vi "Write General Data.vi"(8 "Error In":errorcluster, 9 "AC Advance Step Data":T1 {"Transient Time" format="%.1f ms"; "Transient Site" format="%.0f ¢X"; "Transient Volt" format="%.1f V"; "CF Lo Limit" format="%.2f"; "CF Hi Limit" format="%.2f"; "Q Lo Limit" format="%.0f VAR"; "Q Hi Limit" format="%.0f VAR"; "VA Lo Limit" format="%.0f VA"; "VA Hi Limit" format="%.0f VA"; "PF Lo Limit" format="%.3f"; "PF Hi Limit" format="%.3f"; "P Lo Limit" format="%.0f W"; "P Hi Limit" format="%.0f W"; "AP Lo Limit" format="%.1f A"; "AP Hi Limit" format="%.1f A"; "A Lo Limit" format="%.2f A"; "A Hi Limit" format="%.2f A"; "Delay Time" format="%.1f s"; "£GT" format="%.0f ms"; "£GF" format="%.1f Hz"; "£GV" format="%.1f V"; "Time" format="%.1f s"; "Voltage" format="%.1f V"; "Frequency" format="%.1f Hz"}, 10 "Modbus ID":string, 11 "VISA resource name":refnum<visa-resource-name>) -> (0 "Error Out":errorcluster, 3 "VISA resource name out":refnum<visa-resource-name>)   [LabVIEW 2013]
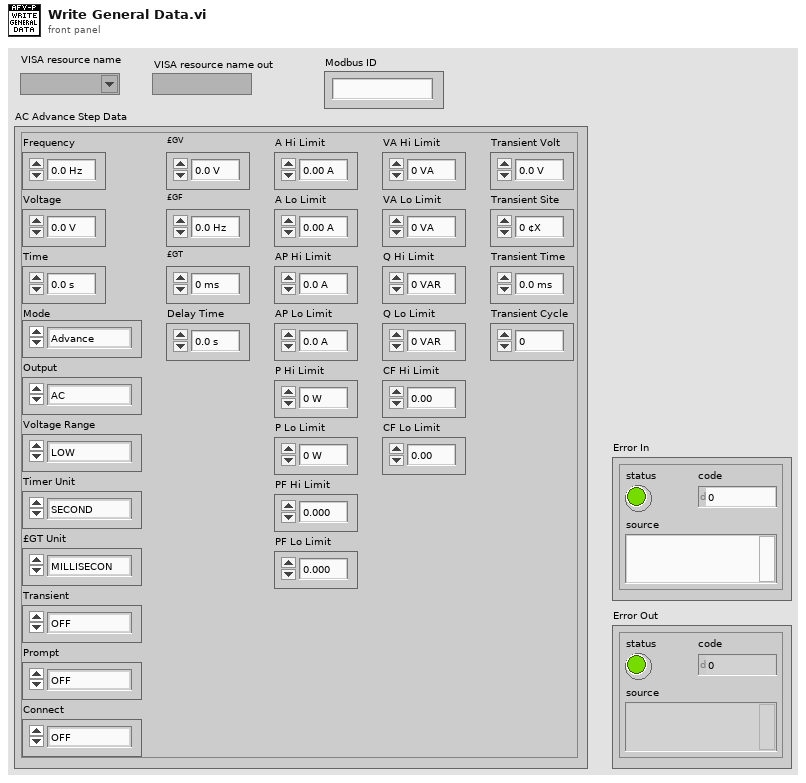
[diagram p1: front panel]
types:
  T1 = cluster{"Frequency":dbl, "Voltage":dbl, "Time":dbl, "Mode":enum16{"Advance", "Basic"}, "Output":enum16{"AC", "DC"}, "Voltage Range":enum16{"LOW", "HIGH", "AUTO"}, "Timer Unit":enum16{"SECOND", "MINUTE", "HOUR"}, "£GT Unit":enum16{"MILLISECON", "SECOND", "CYCLE"}, "Transient":enum16{"OFF", "ON"}, "Prompt":enum16{"OFF", "ON"}, "Connect":enum16{"OFF", "ON"}, "£GV":dbl, "£GF":dbl, "£GT":u16, "Delay Time":dbl, "A Hi Limit":dbl, "A Lo Limit":dbl, "AP Hi Limit":dbl, "AP Lo Limit":dbl, "P Hi Limit":u16, "P Lo Limit":u16, "PF Hi Limit":dbl, "PF Lo Limit":dbl, "VA Hi Limit":u16, "VA Lo Limit":u16, "Q Hi Limit":u16, "Q Lo Limit":u16, "CF Hi Limit":dbl, "CF Lo Limit":dbl, "Transient Volt":dbl, "Transient Site":u16, "Transient Time":dbl, "Transient Cycle":u16}
  T2 = cluster{"Length (High)":string, "Length (Low)":string, "Start Address (High)":string, "Start Address (Middle High)":string, "Start Address (Middle Low)":string, "Start Address (Low)":string}
  T3 = cluster{"ID":string, "Function Code":string, "Length (High)":string, "Length (Low)":string, "Start Address (High)":string, "Start Address (Middle High)":string, "Start Address (Middle Low)":string, "Start Address (Low)":string, "Data":string}
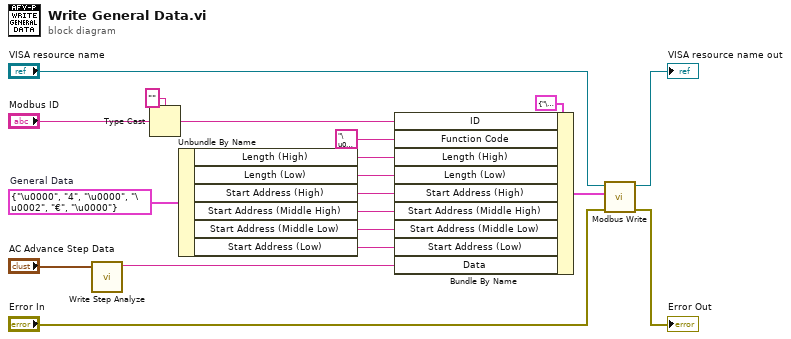
[diagram p0: block diagram]
diagram:
  w12 = T2 {"Length (High)"="\u0000", "Length (Low)"="4", "Start Address (High)"="\u0000", "Start Address (Middle High)"="\u0002", "Start Address (Middle Low)"="€", "Start Address (Low)"="\u0000"}  # General Data
  n1 = call "Write Step Analyze.vi"("AC Advance Step Data"="AC Advance Step Data") -> ("Data"=w4:string)  [unwired: 10 in]
  n2 = Type Cast(type="" ("Binary Data (Hex) 3"), x="Modbus ID") -> (*(type *) &x=w1:string)
  n3 = Unbundle By Name(w12) -> ("Length (High)"=w18:string, "Length (Low)"=w17:string, "Start Address (High)"=w16:string, "Start Address (Middle High)"=w15:string, "Start Address (Middle Low)"=w14:string, "Start Address (Low)"=w13:string)
  n4 = Bundle By Name(cluster=T3 {"ID"="\u0000", "Function Code"="\u0000", "Length (High)"="\u0000", "Length (Low)"="\u0000", "Start Address (High)"="\u0000", "Start Address (Middle High)"="\u0000", "Start Address (Middle Low)"="\u0000", "Start Address (Low)"="\u0000", "Data"=""} ("Write Buffer"), "ID"=w1, "Function Code"="\u0010", "Length (High)"=w18, "Length (Low)"=w17, "Start Address (High)"=w16, "Start Address (Middle High)"=w15, "Start Address (Middle Low)"=w14, "Start Address (Low)"=w13, "Data"=w4) -> (w8:T3)
  n5 = call "Modbus Write.vi"("Error In"="Error In", "Write Buffer"=w8, "VISA resource name"="VISA resource name") -> ("Error Out"=→"Error Out":errorcluster, "VISA resource name out"=→"VISA resource name out":refnum<visa-resource-name>)  [unwired: 7 in]
